vi "Temp ctrl - Disable Ramp.vi"(8 "Error In":errorcluster, 11 "Temp handle":T1={"Connected"=FALSE, "Temp ctrl"={"Gain (P)"=0.0, "Reset (I)"=0.0, "Rate (D)"=0.0, "Stabilization rate"=0.0, "Stabilization delta"=0.0, "Type"=enum."Lake Shore 325", "Custom temp ctrl"={"VISA resource name"=""}, "Lakeshore 325"={"VISA name"="", "Loop"=0, "Heater Range"=1, "Heater Resistance"=0, "Sample sensor"=0, "Fast sensor"=0, "Slow sensor"=0}, "Lakeshore 331"={"VISA name"="", "Loop"=1, "Heater Range"=0, "Sample sensor"=0, "Fast sensor"=0, "Slow sensor"=0}, "Lakeshore 332"={"VISA name"="", "Loop"=1, "Heater Range"=0, "Sample sensor"=0, "Fast sensor"=0, "Slow sensor"=0}, "Lakeshore 335"={"VISA name"="", "Loop"=1, "Sample sensor"=0, "Fast sensor"=0, "Slow sensor"=0, "Heater Range"=0, "Output mode"=enum."Off"}, "Lakeshore 336"={"VISA name"="", "Loop"=1, "Output mode"=enum."Off", "Max current"=1.0, "Heater resistance"=1, "Sample sensor"=1, "Slow sensor"=1, "Fast sensor"=1}}} {"Temp ctrl"."Lakeshore 336"."Fast sensor" items=["Sensor A", "Sensor B", "Sensor C", "Sensor D"]; "Temp ctrl"."Lakeshore 336"."Slow sensor" items=["Sensor A", "Sensor B", "Sensor C", "Sensor D"]; "Temp ctrl"."Lakeshore 336"."Sample sensor" items=["Sensor A", "Sensor B", "Sensor C", "Sensor D"]; "Temp ctrl"."Lakeshore 336"."Heater resistance" items=["25 Ohm"=1, "50 Ohm"=2]; "Temp ctrl"."Lakeshore 336"."Max current" items=["0.707 A"=0.0, "1 A"=1.0, "1.414 A"=1.414, "2 A"=2.0]; "Temp ctrl"."Lakeshore 336"."Loop" items=["Output 1"=1, "Output 2"=2, "Output 3"=3, "Output 4"=4]; "Temp ctrl"."Lakeshore 335"."Heater Range" items=["Off", "Low (On)", "Medium", "High"]; "Temp ctrl"."Lakeshore 335"."Slow sensor" items=["A", "B"]; "Temp ctrl"."Lakeshore 335"."Fast sensor" items=["A", "B"]; "Temp ctrl"."Lakeshore 335"."Sample sensor" items=["A", "B"]; "Temp ctrl"."Lakeshore 335"."Loop" items=["Loop 1"=1, "Loop 2"=2]; "Temp ctrl"."Lakeshore 332"."Slow sensor" items=["A", "B"]; "Temp ctrl"."Lakeshore 332"."Fast sensor" items=["A", "B"]; "Temp ctrl"."Lakeshore 332"."Sample sensor" items=["A", "B"]; "Temp ctrl"."Lakeshore 332"."Heater Range" items=["Off", "Low (0.5W)", "Med (5W)", "High (50W)"]; "Temp ctrl"."Lakeshore 332"."Loop" items=["Loop 1", "Loop 2"]; "Temp ctrl"."Lakeshore 331"."Slow sensor" items=["A", "B"]; "Temp ctrl"."Lakeshore 331"."Fast sensor" items=["A", "B"]; "Temp ctrl"."Lakeshore 331"."Sample sensor" items=["A", "B"]; "Temp ctrl"."Lakeshore 331"."Heater Range" items=["Off", "Low (0.5W)", "Med (5W)", "High (50W)"]; "Temp ctrl"."Lakeshore 331"."Loop" items=["Loop 1", "Loop 2"]; "Temp ctrl"."Lakeshore 325"."Slow sensor" items=["A", "B"]; "Temp ctrl"."Lakeshore 325"."Fast sensor" items=["A", "B"]; "Temp ctrl"."Lakeshore 325"."Sample sensor" items=["A", "B"]; "Temp ctrl"."Lakeshore 325"."Heater Resistance" items=["25 Ohm"=1, "50 Ohm"=2]; "Temp ctrl"."Lakeshore 325"."Heater Range" items=["Off", "Low (loop 1) or On (loop 2)", "High (loop 1)"]; "Temp ctrl"."Lakeshore 325"."Loop" items=["Loop 1"=1, "Loop 2"=2]}) -> (0 "Error Out":errorcluster)   [LabVIEW 2019]
doc: "Disables ramp mode of the temperature controller"
uses:
  Type defs/Temp handle Type Def.ctl
  Type defs/Temp ctrl Type Def.ctl
  Custom devices/Custom temp ctrl settings.ctl
  <instrlib>/Lake Shore 325/Lake Shore 325.lvlib
  <instrlib>/Lake Shore Cryotronics 331/Lake Shore Cryotronics 331.lvlib
  <instrlib>/Lake Shore Cryotronics 332/Lake Shore Cryotronics 332.lvlib
  <instrlib>/Lake Shore 335/Lake Shore 335.lvlib
  <instrlib>/Lake Shore 336/Lake Shore 336.lvlib
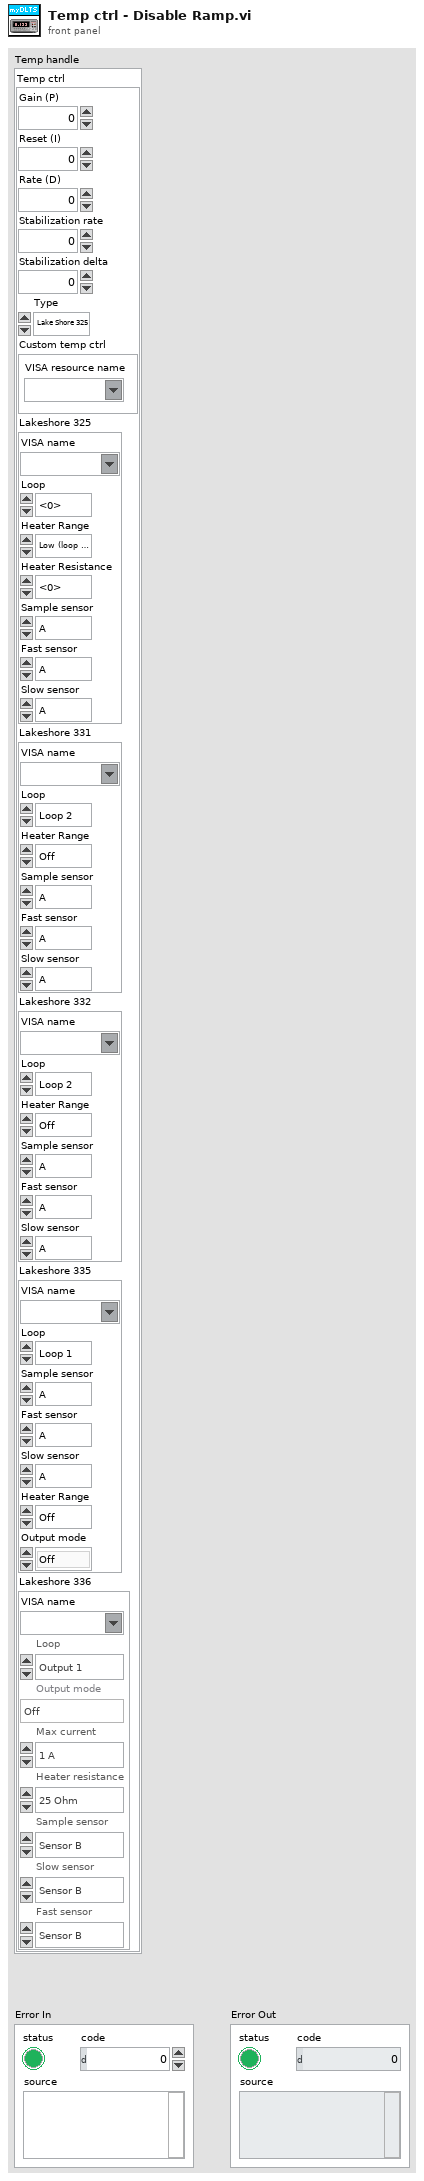
[diagram p1: front panel]
types:
  T1 = typedef "Temp handle Type Def.ctl" = cluster{"Connected":bool, "Temp ctrl":T2}
  T2 = typedef "Temp ctrl Type Def.ctl" = cluster{"Gain (P)":dbl, "Reset (I)":dbl, "Rate (D)":dbl, "Stabilization rate":dbl, "Stabilization delta":dbl, "Type":enum16{"Custom", "Lake Shore 325", "Lake Shore 331", "Lake Shore 332", "Lake Shore 335", "Lake Shore 336"}, "Custom temp ctrl":T3, "Lakeshore 325":cluster{"VISA name":refnum<visa-resource-name>, "Loop":u16, "Heater Range":u16, "Heater Resistance":u16, "Sample sensor":u16, "Fast sensor":u16, "Slow sensor":u16}, "Lakeshore 331":cluster{"VISA name":refnum<visa-resource-name>, "Loop":u16, "Heater Range":u16, "Sample sensor":u16, "Fast sensor":u16, "Slow sensor":u16}, "Lakeshore 332":cluster{"VISA name":refnum<visa-resource-name>, "Loop":u16, "Heater Range":u16, "Sample sensor":u16, "Fast sensor":u16, "Slow sensor":u16}, "Lakeshore 335":cluster{"VISA name":refnum<visa-resource-name>, "Loop":u16, "Sample sensor":u16, "Fast sensor":u16, "Slow sensor":u16, "Heater Range":u16, "Output mode":enum16{"Off", "Closed Loop PID", "Zone", "Open Loop", "Monitor Out", "Warmup Supply"}}, "Lakeshore 336":cluster{"VISA name":refnum<visa-resource-name>, "Loop":u16, "Output mode":enum16{"Off", "Closed Loop PID", "Zone", "Open Loop"}, "Max current":dbl, "Heater resistance":u16, "Sample sensor":u16, "Slow sensor":u16, "Fast sensor":u16}}
  T3 = typedef "Custom temp ctrl settings.ctl" = cluster{"VISA resource name":refnum<visa-resource-name>}
  T4 = enum16{"Custom", "Lake Shore 325", "Lake Shore 331", "Lake Shore 332", "Lake Shore 335", "Lake Shore 336"}
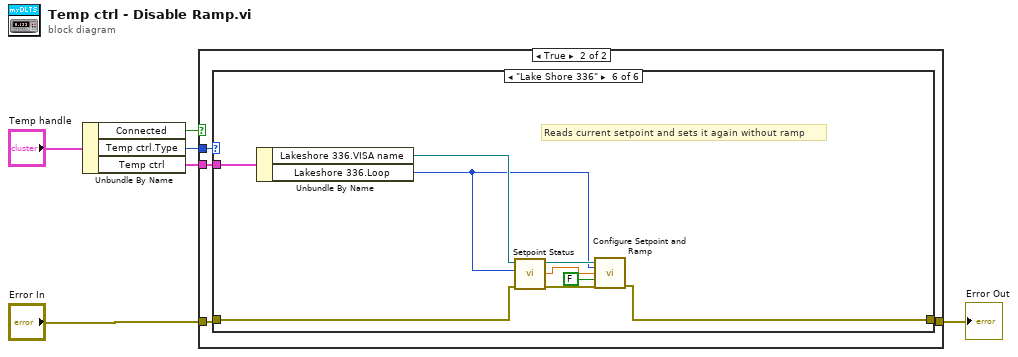
[diagram p0: block diagram]
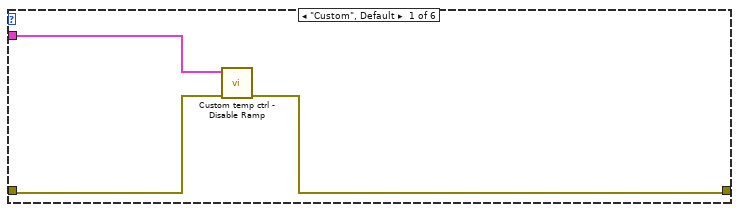
[diagram p3: hidden frame]
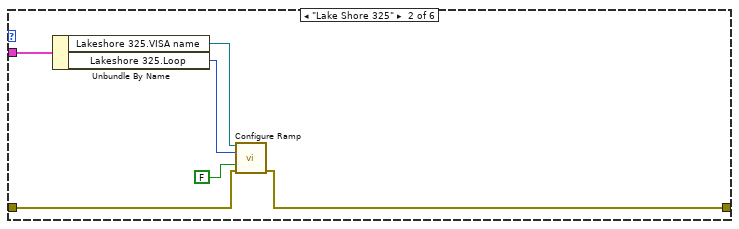
[diagram p4: hidden frame]
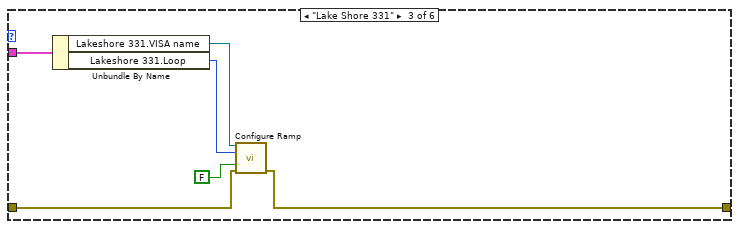
[diagram p5: hidden frame]
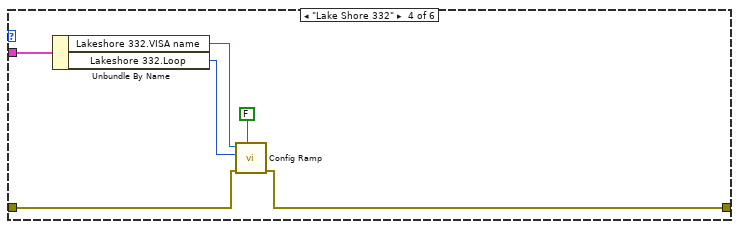
[diagram p6: hidden frame]
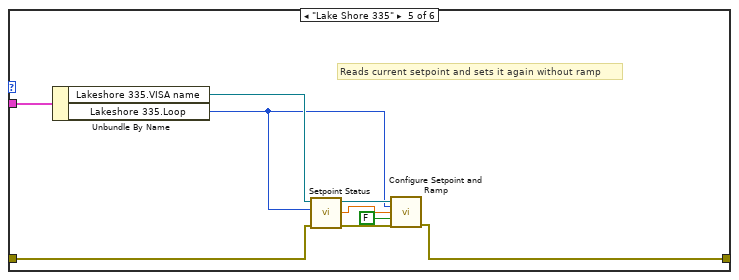
[diagram p7: hidden frame]
diagram:
  n1 = Unbundle By Name("Temp handle") -> ("Connected"=w6:bool, "Temp ctrl.Type"=w5:T4, "Temp ctrl"=w3:T2)
  n2 = case shown="True" w6 {
    tunnel: w5 -> [_ w11]
    tunnel: w3 -> [_ w10]
    tunnel: "Error In" -> [w7 w9]
    tunnel: [w7 w8] -> w1
    frame False {
    }
    frame True {
      n3 = case shown="\"Lake Shore 336\"" w11 {
        tunnel: w10 -> [w12 w20 w26 w32 w41 w50]
        tunnel: w9 -> [w14 w19 w25 w31 w35 w44]
        tunnel: [w13 w15 w21 w27 w34 w43] -> w8
        frame "Custom", Default {
          n4 = call "Custom temp ctrl - Disable Ramp.vi"("Error In"=w14, "Temp ctrl"=w12) -> ("Error Out"=w13:errorcluster)  [unwired: 9 in]
        }
        frame "Lake Shore 325" {
          n5 = Unbundle By Name(w20) -> ("Lakeshore 325.VISA name"=w17:refnum<visa-resource-name>, "Lakeshore 325.Loop"=w18:u16)
          n6 = call <instrlib>:"Configure Ramp.vi"("VISA resource name"=w17, "Loop (1:Loop 1)"=w18, "Setpoint Ramp (F: Off)"=FALSE, "error in (no error)"=w19) -> ("error out"=w15:errorcluster)  [unwired: 10 in, 1 out]
        }
        frame "Lake Shore 331" {
          n7 = Unbundle By Name(w26) -> ("Lakeshore 331.VISA name"=w23:refnum<visa-resource-name>, "Lakeshore 331.Loop"=w24:u16)
          n8 = call <instrlib>:"Configure Ramp.vi"("VISA resource name"=w23, "Loop (0: 1)"=w24, "Ramping On/Off (F: Off)"=FALSE ("Setpoint Ramp (F: Off)"), "error in (no error)"=w25) -> ("error out"=w21:errorcluster)  [unwired: 10 in, 1 out]
        }
        frame "Lake Shore 332" {
          n9 = Unbundle By Name(w32) -> ("Lakeshore 332.VISA name"=w29:refnum<visa-resource-name>, "Lakeshore 332.Loop"=w30:u16)
          n10 = call <instrlib>:"Config Ramp.vi"("Ramping On-Off (F: Off)"=FALSE ("Setpoint Ramp (F: Off)"), "error in (no error)"=w31, "Loop (0: 1)"=w30, "VISA resource name"=w29) -> ("error out"=w27:errorcluster)  [unwired: 6 in, 1 out]
        }
        frame "Lake Shore 335" {
          # "Reads current setpoint and sets it again without ramp"
          n11 = Unbundle By Name(w41) -> ("Lakeshore 335.VISA name"=w36:refnum<visa-resource-name>, "Lakeshore 335.Loop"=w33:u16)
          n12 = call <instrlib>:"Setpoint Status.vi"("error in (no error)"=w35, "Output (1:1)"=w33, "VISA resource name"=w36) -> ("error out"=w40:errorcluster, "Setpoint"=w38:dbl, "VISA resource name out"=w37:refnum<visa-resource-name>)  [unwired: 6 in]
          n13 = call <instrlib>:"Configure Setpoint and Ramp.vi"("VISA resource name"=w37, "Output's Control Loop (1:1)"=w33, "Setpoint (0.0000)"=w38, "Enable Setpoint Ramping (F: Off)"=FALSE, "error in (no error)"=w40) -> ("error out"=w34:errorcluster)  [unwired: 9 in, 1 out]
        }
        frame "Lake Shore 336" {
          # "Reads current setpoint and sets it again without ramp"
          n14 = Unbundle By Name(w50) -> ("Lakeshore 336.VISA name"=w45:refnum<visa-resource-name>, "Lakeshore 336.Loop"=w42:u16)
          n15 = call <instrlib>:"Setpoint Status.vi"("error in (no error)"=w44, "Output (1:1)"=w42, "VISA resource name"=w45) -> ("error out"=w49:errorcluster, "Setpoint"=w47:dbl, "VISA resource name out"=w46:refnum<visa-resource-name>)  [unwired: 6 in]
          n16 = call <instrlib>:"Configure Setpoint and Ramp.vi"("VISA resource name"=w46, "Output's Control Loop (1:1)"=w42, "Setpoint (0.00000)"=w47, "Setpoint Ramping \nEnable (F: Off)"=FALSE ("Enable Setpoint Ramping (F: Off)"), "error in (no error)"=w49) -> ("error out"=w43:errorcluster)  [unwired: 9 in, 1 out]
        }
      }
    }
  }
  "Error Out" <- w1
